vi "Create Message Queue.vi"(8 "Error In":errorcluster) -> (0 "Error Out":errorcluster, 3 "Message Queue":refnum<queue>)   [LabVIEW 2017, in "Eulogy.lvlib" / "Bookmark Manager.lvlib"]
uses:
  Bookmark Manager.lvlib
  Message.ctl
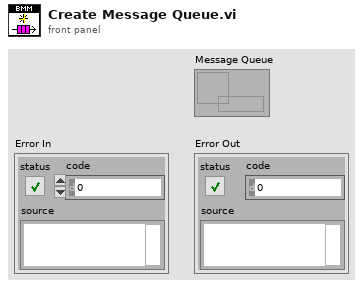
[diagram p1: front panel]
types:
  T1 = typedef "Eulogy.lvlib/Bookmark Manager.lvlib/Message.ctl" = cluster{"Command":string, "Data":variant}
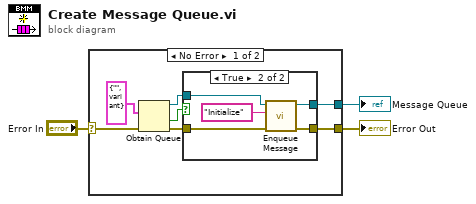
[diagram p0: block diagram]
diagram:
  n1 = case shown="No Error" "Error In" {
    selector: "Error In" -> [w6 w18]
    tunnel: [w5 w18] -> w2
    tunnel: [w4 _] -> w1
    frame No Error {
      n2 = Obtain Queue(element data type=T1 {"Command"="", "Data"=variant} ("Message"), error in (no error)=w6) -> (queue out=w8:refnum<queue>, created new?=w9:bool, error out=w7:errorcluster)  [unwired: 3 in]
      n3 = case shown="True" w9 {
        tunnel: w8 -> [w11 w17]
        tunnel: w7 -> [w12 w16]
        tunnel: [w12 w14] -> w5
        tunnel: [w11 w13] -> w4
        frame False {
        }
        frame True {
          n4 = call "Enqueue Message.vi"("Error In"=w16, "Command"="Initialize", "Message Queue In"=w17) -> ("Error Out"=w14:errorcluster, "Message Queue Out"=w13:refnum<queue>)  [unwired: 7 in]
        }
      }
    }
    frame Error {
    }
  }
  "Error Out" <- w2
  "Message Queue" <- w1
